vi "AMWave.vi"(9 "AM Wave Parameters":T1, 10 "Digitizing Parameters":T2) -> (2 "AM Wave":cluster{"t":dbl[], "x":dbl[]})   [LabVIEW 2014]
doc: "Problem DIY)\n\nThis VI produces an AM modulated signal from a series of input parameter. And made into a VI subfunction."
uses:
  <vilib>/imath/engines/lvmath2/RunTimeEngine/Managers/WorkSpace/UID Generator.vi
  <vilib>/imath/engines/lvmath2/RunTimeEngine/RunTimeType/NIMS_RunTimeType_From StrictType (excl LVString).vi
  <instcachedir>/0/NIMS_RunTimeType_From StrictType (excl LVString)_15A5391EEA9C4AACB9955AC755B83D29.lvgen/NIMS_RunTimeType_From StrictType (excl LVString)_15A5391EEA9C4AACB9955AC755B83D29_000.vi
  <vilib>/imath/engines/lvmath2/RunTimeEngine/LocalVariableDefStatement/MC_LocalVariableDefStatement_Display.vi
  <vilib>/imath/engines/lvmath2/RunTimeEngine/RangeToken/NIMS_Range.vi
  <instcachedir>/0/NIMS_Range_9BCE657718DF4976A877346C61F22738.lvgen/NIMS_Range_9BCE657718DF4976A877346C61F22738_000.vi
  <vilib>/imathl/engines/lvmath/Functions/Error Handling/Create Error.vi
  <vilib>/imath/engines/lvmath2/RunTimeEngine/ArithmeticOperatorToken/NIMS_ArithmeticOperator_times.vi
  <instcachedir>/0/NIMS_ArithmeticOperator_times_2EFF5B13FCA4492A81D59089AD809F54.lvgen/NIMS_ArithmeticOperator_times_2EFF5B13FCA4492A81D59089AD809F54_000.vi
  <vilib>/imath/engines/lvmath2/RunTimeEngine/Managers/SymbolTable/Clear UID.vi
  <vilib>/imath/engines/lvmath2/RunTimeEngine/NodeEndStatement/NIMS_NodeEndStatement_Output.vi
  <instcachedir>/0/NIMS_NodeEndStatement_Output_53EC0D466D134D7ABD903AC30B43404B.lvgen/NIMS_NodeEndStatement_Output_53EC0D466D134D7ABD903AC30B43404B_005.vi
  <vilib>/imath/engines/lvmath2/RunTimeEngine/ErrorHandling/NIMS_Finalize Error.vi
  <vilib>/imath/engines/lvmath2/RunTimeEngine/Managers/SymbolTable/NIMS_WorkSpace.lvlib
panel:
  out "XY Graph":cluster{"t":dbl[], "x":dbl[]}(graph)
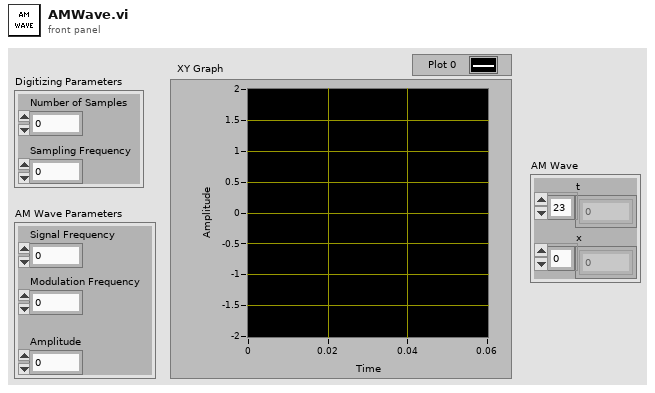
[diagram p1: front panel]
types:
  T1 = cluster{"Signal Frequency":dbl, "Modulation Frequency":dbl, "Amplitude":dbl}
  T2 = cluster{"Number of Samples":dbl, "Sampling Frequency":dbl}
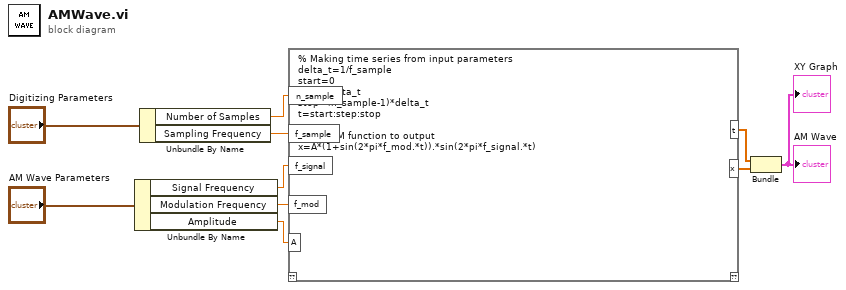
[diagram p0: block diagram]
diagram:
  n1 = Unbundle By Name("AM Wave Parameters") -> ("Signal Frequency"=w4:dbl, "Modulation Frequency"=w3:dbl, "Amplitude"=w2:dbl)
  n2 = Unbundle By Name("Digitizing Parameters") -> ("Number of Samples"=w6:dbl, "Sampling Frequency"=w5:dbl)
  n3 = mathscript code="% Making time series from input parameters\ndelta_t=1/f_sample\nstart=0\nstep=delta_t\nstop=(n_sample-1)*delta_t\nt=start:step:stop\n\n% The AM function to output\nx=A*(1+sin(2*pi*f_mod.*t)).*sin(2*pi*f_signal.*t)"("n_sample"=w6, "f_sample"=w5, "f_signal"=w4, "f_mod"=w3, "A"=w2) -> ("t"=w10:dbl[], "x"=w9:dbl[])  [unwired: 1 in, 1 out]
  n4 = Bundle("t"=w10, "x"=w9) -> (→"XY Graph" →"AM Wave":cluster{"t":dbl[], "x":dbl[]})  [unwired: 1 in]
